vi "Integration Test Launcher-VIM.vi"() -> ()   [LabVIEW 2019]
doc: "<License>\nCopyright © 2020 Tymphany, LLC | All rights reserved\nwww.Tymphany.com\nHuijun <Huijun.Guo@Tymphany.com>\n</License>"
uses:
  <vilib>/gpm_packages/@cs/example/Integration Test/ConcreteViewModel/ConcreteViewModel.lvclass
  C:/Program Files/National Instruments/LabVIEW 2019/vi.lib/gpm_packages/@cs/mva-core/Source/IObserver/IObserver/IObserver.lvclass
  C:/Program Files/National Instruments/LabVIEW 2019/vi.lib/gpm_packages/@cs/mva-viewable/Source/IViewModel/IViewModel/IViewModel.lvclass
  C:/Program Files/National Instruments/LabVIEW 2019/vi.lib/ActorFramework/Actor/Actor.lvclass
  <vilib>/gpm_packages/@cs/example/Integration Test/ValueChangeEventProducer/ValueChangeEventProducer.lvclass
  C:/Program Files/National Instruments/LabVIEW 2019/vi.lib/gpm_packages/@cs/mva-viewable/Source/IViewable/IViewable/IViewable.lvclass
  <vilib>/gpm_packages/@cs/example/Integration Test/BasicAutoRegistrationView/BasicAutoRegistrationView.lvclass
  <vilib>/gpm_packages/@cs/example/Integration Test/ActorAutoRegistrationView/EventHandlingActor.lvclass
  <vilib>/gpm_packages/@cs/mva-viewable/Source/IViewable/IViewable/View Position Enum.ctl
  <vilib>/gpm_packages/@cs/example/Integration Test/ConcreteModel/ConcreteModel.lvclass
  C:/Program Files/National Instruments/LabVIEW 2019/vi.lib/gpm_packages/@cs/mva-core/Source/IModel/IModel/IModel.lvclass
  <vilib>/gpm_packages/@cs/example/Integration Test/TreeActor/TreeActor.lvclass
  <vilib>/gpm_packages/@cs/example/Integration Test/MCListboxActor/MCListboxActor.lvclass
  <vilib>/Utility/miscctls.llb/LVPointTypeDef.ctl
  <vilib>/gpm_packages/@cs/mva-core/Source/MonitoredMediator/MonitoredMediator/MonitoredMediator.lvclass
  C:/Program Files/National Instruments/LabVIEW 2019/vi.lib/gpm_packages/@cs/mva-core/Source/IMediator/IMediator/IMediator.lvclass
  <vilib>/ActorFramework/Message Enqueuer/Message Priority.ctl
  <vilib>/gpm_packages/@cs/example/Integration Test/BasicTerminalBinding/BasicTerminalBinding.lvclass
  <vilib>/gpm_packages/@cs/example/Integration Test/MultiSubscriber/MultiSubscriber.lvclass
  <vilib>/gpm_packages/@cs/example/Integration Test/BasicChartBinding/BasicChartBinding.lvclass
  <vilib>/gpm_packages/@cs/BusMonitor/ListboxBusMonitor/ListboxBusMonitor/ListboxBusMonitor.lvclass/ListboxBusMonitor.ctl
  <vilib>/gpm_packages/@cs/mva-core/Source/MonitoredMediator/MonitoredMediator/MonitoredMediator.lvclass/MonitoredMediator.ctl
  <vilib>/gpm_packages/@cs/event-logger/Source/Composed Log/LoggerReference/LoggerReference.lvclass/LoggerReference.ctl
  <vilib>/gpm_packages/@cs/mva-core/Source/IObserver/IObserver/IObserver.lvclass/IObserver.ctl
  <vilib>/gpm_packages/@cs/mva-core/Source/IMediator/IMediator/IMediator.lvclass/IMediator.ctl
  <vilib>/gpm_packages/@cs/mva-viewable/Source/IViewModel/IViewModel/IViewModel.lvclass/IViewModel.ctl
  <vilib>/gpm_packages/@cs/mva-viewable/Source/IViewManager/IViewManager Messages/Launch Nested Views Msg/Launch Nested Views Msg.lvclass/Launch Nested Views Msg.ctl
  <vilib>/gpm_packages/@cs/mva-viewable/Source/IViewManager/IViewManager/IViewManager.lvclass/IViewManager.ctl
  <vilib>/gpm_packages/@cs/mva-viewable/Source/IViewable/IViewable Messages/Open Front Panel Msg/Open Front Panel Msg.lvclass/Open Front Panel Msg.ctl
  <vilib>/ActorFramework/Message Enqueuer/Message Enqueuer.lvclass/Message Enqueuer.ctl
  <vilib>/gpm_packages/@cs/mva-viewable/Source/IViewable/IViewable Messages/Set Minimum Panel Size Msg/Set Minimum Panel Size Msg.lvclass/Set Minimum Panel Size Msg.ctl
  <vilib>/gpm_packages/@cs/event-logger/Source/ConsoleView/ConsoleInterface/ConsoleSession.lvclass/ConsoleSession.ctl
  6a041f87-186a-4215-a0f2-d15be5a5cb52.vi
  6765fa55-9b8c-4fa0-b8dd-700a6345a818.vi
  <vilib>/gpm_packages/@cs/mva-core/Source/MonitoredMediator/MonitoredMediator/Private Write BusMonitors.vi
  6765fa55-9b8c-4fa0-b8dd-700a6345a818.vi/128054e4-2619-4af6-9b08-2daa041eaefc.vi
  <vilib>/gpm_packages/@cs/mva-core/Source/IObserver/IObserver/Configure Observer Logging.vi
  <vilib>/gpm_packages/@cs/mva-viewable/Source/IViewModel/IViewModel/Write Startup Model-View Configuration.vi
  <vilib>/gpm_packages/@cs/mva-core/Source/IMediator/IMediator/Configure Mediator.vi
  <vilib>/ActorFramework/Message Enqueuer/Enqueue.vi
  <vilib>/gpm_packages/@cs/event-logger/Source/Composed Log/LoggerReference/Return Aggregate Queues.vi
  <vilib>/gpm_packages/@cs/event-logger/Source/Composed Log/LoggerReference/Add Aggregate Log.vi
  6765fa55-9b8c-4fa0-b8dd-700a6345a818.vi/128054e4-2619-4af6-9b08-2daa041eaefc.vi/dc909d2e-44c5-409a-9135-51858d3a7512.vi
  <vilib>/gpm_packages/@cs/mva-viewable/Source/IViewManager/IViewManager Messages/Launch Nested Views Msg/Pack Launch Nested Views Msg.vi
  <vilib>/gpm_packages/@cs/mva-viewable/Source/IViewManager/IViewManager/Write Startup Launch Nested Views Msg.vi
  <vilib>/gpm_packages/@cs/event-logger/Source/Composed Log/LoggerReference/Send Add Sink.vi
  <vilib>/gpm_packages/@cs/ViewManager/source/QuadViewManager/QuadViewManager.lvclass
  C:/Program Files/National Instruments/LabVIEW 2019/vi.lib/gpm_packages/@cs/mva-viewable/Source/IViewManager/IViewManager/IViewManager.lvclass
  <vilib>/gpm_packages/@cs/ViewManager/source/BoundViewManager/BoundViewManager.lvclass
  <vilib>/gpm_packages/@cs/ViewManager/source/TabbedViewManager/TabbedViewManager.lvclass
  <vilib>/gpm_packages/@cs/mva-viewable/Source/IViewManager/IViewManager/IViewManager.lvclass
  <vilib>/gpm_packages/@cs/event-logger/Source/ConsoleView/Sink/ConsoleSink.lvclass
  C:/Program Files/National Instruments/LabVIEW 2019/vi.lib/gpm_packages/@cs/event-logger/Source/Composed Log/Log Sink/Log Sink.lvclass
  <vilib>/gpm_packages/@cs/ViewManager/source/LeftListboxViewManager/LeftListboxViewManager.lvclass
  <vilib>/gpm_packages/@cs/mva-viewable/Source/IViewModel/IViewModel/IViewModel.lvclass
  <vilib>/gpm_packages/@cs/mva-viewable/Source/IViewable/IViewable Messages/Open Front Panel Msg/Open Front Panel Msg.lvclass
  C:/Program Files/National Instruments/LabVIEW 2019/vi.lib/ActorFramework/Message/Message.lvclass
  <vilib>/gpm_packages/@cs/mva-viewable/Source/IViewable/IViewable Messages/Set Minimum Panel Size Msg/Set Minimum Panel Size Msg.lvclass
  <vilib>/gpm_packages/@cs/event-logger/Source/Composed Log/Application Logger/Launch Worker Loop.vi
  <vilib>/gpm_packages/@cs/event-logger/Source/Composed Log/LoggerReference/Initialize Logger Instance.vi
  <vilib>/ActorFramework/Message Priority Queue/Priority Enqueue.vi
  <vilib>/gpm_packages/@cs/BusMonitor/ListboxBusMonitor/ListboxBusMonitor/ListboxBusMonitor.lvclass
  <vilib>/gpm_packages/@cs/event-logger/Source/Composed Log/LoggerReference/LoggerReference.lvclass
  <vilib>/gpm_packages/@cs/event-logger/Source/Composed Log/IErrorFormat/IErrorFormat.lvclass
  <vilib>/gpm_packages/@cs/event-logger/Source/Composed Log/Log Sink/Log Sink.lvclass
  <vilib>/gpm_packages/@cs/mva-viewable/Source/IViewable/IApplicationStyle/IApplicationStyle.lvclass
  <vilib>/gpm_packages/@cs/mva-viewable/Source/IViewManager/IViewManager Messages/Launch Nested Views Msg/Launch Nested Views Msg.lvclass
  <vilib>/ActorFramework/Actor/Actor.lvclass
  <vilib>/gpm_packages/@cs/mva-viewable/Source/IViewable/IViewable/IViewable.lvclass
  <vilib>/ActorFramework/Message Enqueuer/Message Enqueuer.lvclass
  <vilib>/gpm_packages/@cs/event-logger/Source/ConsoleView/ConsoleInterface/ConsoleSession.lvclass
panel:
  out "error out":errorcluster
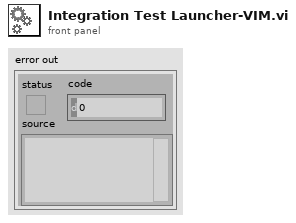
[diagram p1: front panel]
types:
  T1 = typedef "Actor Framework.lvlib/Message Enqueuer.lvclass/Message Priority.ctl" = enum16{"Low", "Normal", "High"}
  T2 = typedef "LVPointTypeDef.ctl" = cluster{"Horizontal":i16, "Vertical":i16}
  T3 = typedef "IViewable.lvlib/IViewable.lvclass/View Position Enum.ctl" = enum16{"Centered", "Maximized", "Minimized", "Custom", "Unchanged"}
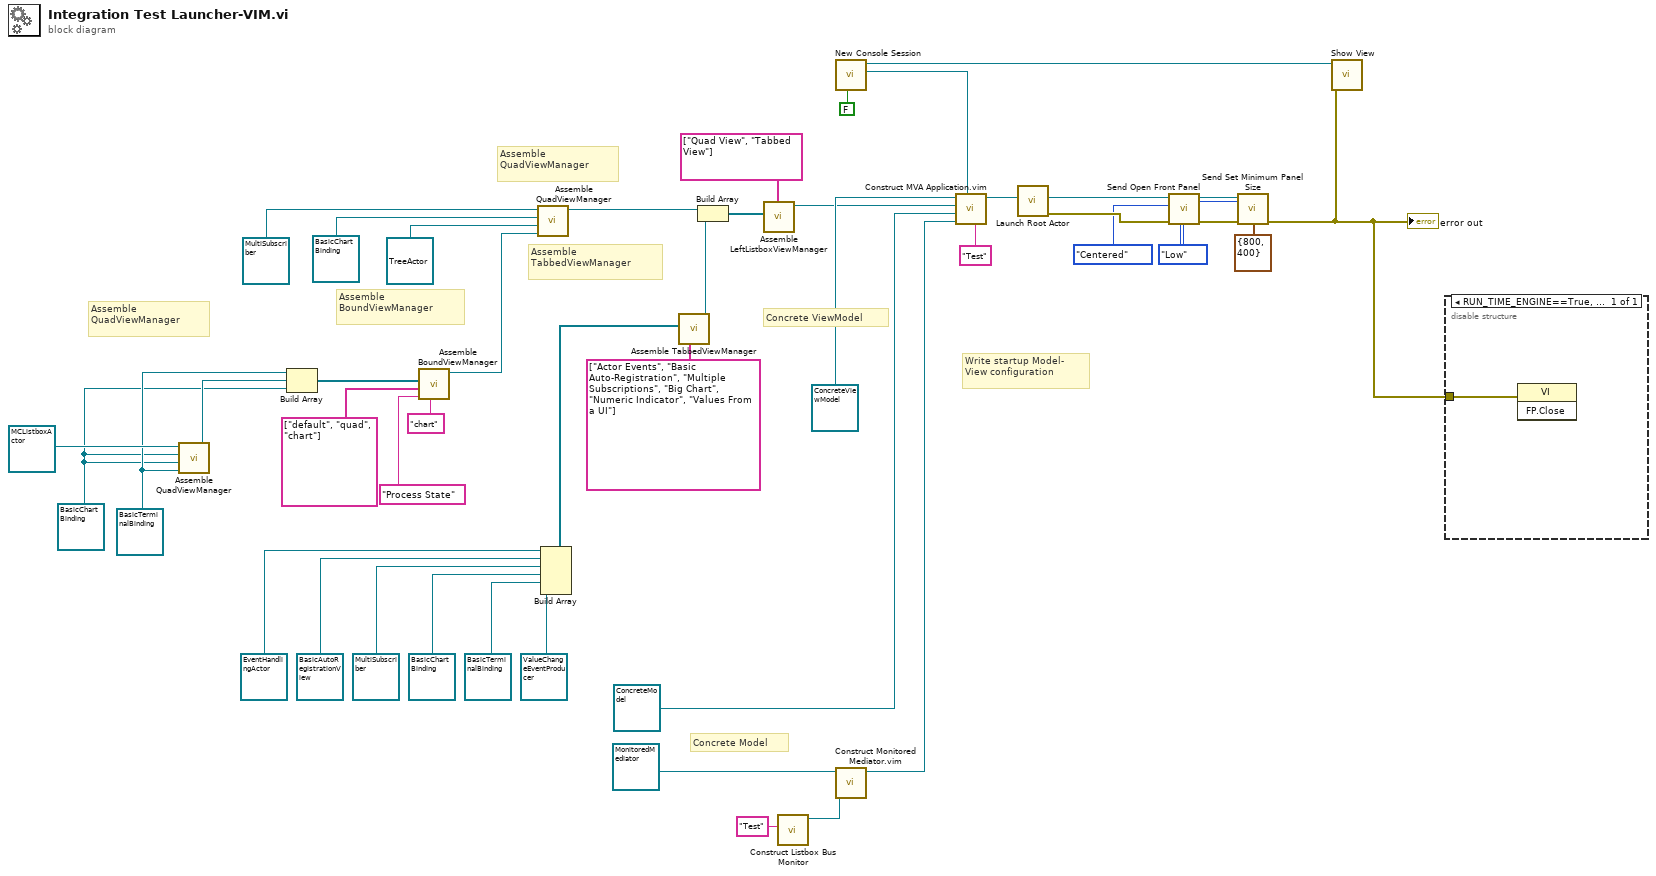
[diagram p0: block diagram]
diagram:
  w14 = Message_Priority."Low" ("Message Priority (Normal)")
  w13 = refnum<class "BasicTerminalBinding.lvclass"> refnum ("TestActors.lvlib:NumericCounter.lvclass")
  w8 = refnum<class "BasicChartBinding.lvclass"> refnum ("TestActors.lvlib:RandomDataChart.lvclass")
  # "Write startup Model-\nView configuration"
  # "Assemble\nBoundViewManager"
  # "Assemble\nQuadViewManager"
  # "Assemble\nQuadViewManager"
  # "Assemble\nTabbedViewManager"
  # "Concrete Model"
  # "Concrete ViewModel"
  n1 = call <vilib>:"Assemble QuadViewManager.vi"("Bottom-Right View"=w13, "Bottom-Left View"=w8, "Top-Right View"=w8, "Top-Left View"=refnum<class "MCListboxActor.lvclass"> refnum ("TestViewables.lvlib:MCListboxActor.lvclass")) -> ("QuadViewManager out"=w29:refnum<class "QuadViewManager.lvclass">)  [unwired: 7 in]
  n2 = Build Array(w13, w29, w8) -> (w28:refnum<class "IViewable.lvclass">[])
  n3 = call <vilib>:"Assemble BoundViewManager.vi"("Startup View Name (\"\"=None)"="chart" ("Startup View Name (\"\"=None)"), "Selector String Name"="Process State", "Viewable Names"=string[] ["default", "quad", "chart"] ("Insertion Names"), "Bound Viewables"=w28) -> ("BoundViewManager Out"=w30:refnum<class "BoundViewManager.lvclass">)  [unwired: 7 in]
  n4 = call <vilib>:"Assemble QuadViewManager.vi"("Bottom-Right View"=w30, "Bottom-Left View"=refnum<class "TreeActor.lvclass"> refnum ("TestViewables.lvlib:TreeActor.lvclass"), "Top-Right View"=refnum<class "BasicChartBinding.lvclass"> refnum ("TestActors.lvlib:RandomDataChart.lvclass"), "Top-Left View"=refnum<class "MultiSubscriber.lvclass"> refnum ("TestActors.lvlib:ButtonPanel.lvclass")) -> ("QuadViewManager out"=w37:refnum<class "QuadViewManager.lvclass">)  [unwired: 7 in]
  n5 = Build Array(refnum<class "EventHandlingActor.lvclass"> refnum ("ActorAutoRegPanel"), refnum<class "BasicAutoRegistrationView.lvclass"> refnum ("AutoRegPanel"), refnum<class "MultiSubscriber.lvclass"> refnum ("TestActors.lvlib:ButtonPanel.lvclass"), refnum<class "BasicChartBinding.lvclass"> refnum ("TestActors.lvlib:RandomDataChart.lvclass"), refnum<class "BasicTerminalBinding.lvclass"> refnum ("TestActors.lvlib:NumericCounter.lvclass"), refnum<class "ValueChangeEventProducer.lvclass"> refnum ("TestActors.lvlib:NumericInputs.lvclass")) -> (w43:refnum<class "IViewable.lvclass">[])
  n6 = call <vilib>:"Assemble TabbedViewManager.vi"("View Names"=string[] ["Actor Events", "Basic Auto-Registration", "Multiple Subscriptions", "Big Chart", "Numeric Indicator", "Values From a UI"] ("View Labels"), "Views"=w43) -> ("TabbedViewManager Out"=w41:refnum<class "TabbedViewManager.lvclass">)  [unwired: 9 in]
  n7 = Build Array(w37, w41) -> (w42:refnum<class "IViewManager.lvclass">[])
  n8 = call <vilib>:"Assemble LeftListboxViewManager.vi"("View Names"=string[] ["Quad View", "Tabbed View"] ("View Labels"), "Views"=w42) -> ("LeftListboxViewManager Out"=w19:refnum<class "LeftListboxViewManager.lvclass">)  [unwired: 9 in]
  n9 = call <vilib>:"Construct Listbox Bus Monitor.vi"("Show Panel Boolean Name"="Test") -> ("ListboxBusMonitor out"=w2:refnum<class "ListboxBusMonitor.lvclass">)  [unwired: 10 in]
  n10 = call <vilib>:"New Console Session.vi"("Persist After Shutdown?(F)"=FALSE) -> ("ConsoleSink out"=w4:refnum<class "ConsoleSink.lvclass">, "ConsoleSession out"=w6:refnum<class "ConsoleSession.lvclass">)  [unwired: 8 in, 1 out]
  n11 = call "Construct Monitored Mediator.vim"("Startup Bus Monitor(s)"=w2, "MonitoredMediator in"=refnum<class "MonitoredMediator.lvclass"> refnum ("MonitoredMediator.lvlib:MonitoredMediator.lvclass")) -> ("MonitoredMediator out"=w16:refnum<class "MonitoredMediator.lvclass">)  [unwired: 9 in]
  n12 = call "Construct MVA Application.vim"("Framework Instance Alias"="Test", "Event Log Sink(s)"=w4, "Mediator Type"=w16, "Model Type"=refnum<class "ConcreteModel.lvclass"> refnum ("TopLevelApplication.lvlib:ConcreteModel.lvclass"), "Startup View Configuration"=w19, "IViewModel In"=refnum<class "ConcreteViewModel.lvclass"> refnum ("TopLevelApplication.lvlib:TopLevelApplication.lvclass")) -> ("IViewModel Out"=w44:refnum<class "ConcreteViewModel.lvclass">)  [unwired: 5 in]
  n13 = call <vilib>:"Launch Root Actor.vi"("Actor"=w44) -> ("error out"=w32:errorcluster, "Actor's Enqueuer"=w34:refnum<class "Message Enqueuer.lvclass">)  [unwired: 9 in]
  n14 = call <vilib>:"Send Open Front Panel.vi"("Message Priority (Normal)"=w14, "error in (no error)"=w32, "Position"=View_Position_Enum."Centered", "Message Enqueuer"=w34) -> ("error out"=w33:errorcluster, "Message Enqueuer out"=w22:refnum<class "Message Enqueuer.lvclass">)  [unwired: 6 in]
  n15 = call <vilib>:"Send Set Minimum Panel Size.vi"("Message Priority (Normal)"=w14, "error in (no error)"=w33, "Minimum Size"=T2 {"Horizontal"=800, "Vertical"=400}, "Message Enqueuer"=w22) -> ("error out"=w3:errorcluster)  [unwired: 6 in, 1 out]
  "error out" <- w3
  n16 = call <vilib>:"Show View.vi"("error in (no error)"=w3, "ConsoleInterface in"=w6) -> ()  [unwired: 8 in, 2 out]
  n17 = disable-structure shown="RUN_TIME_ENGINE==True, Default" {
    disable-tunnel: w3 -> [w45]
    frame condition #0 (active) {
      n18 = invoke class="VI" method="FP.Close"(error in=w45) -> ()  [unwired: 2 in, 3 out]
    }
  }
